vi "Client_Create.vi"(5 "Engine Factory":refnum<class "EngineFactory.lvclass">, 11 "Error In":errorcluster) -> (4 "reference out":refnum<class "Client.lvclass">, 15 "Error Out":errorcluster)   [LabVIEW 2024, in "Client.lvclass"]
uses:
  Client.lvclass/Client.ctl
  Client.lvclass
  Factory Folder/EngineFactory/EngineFactory.lvclass
panel:
  # "Connector Pane"
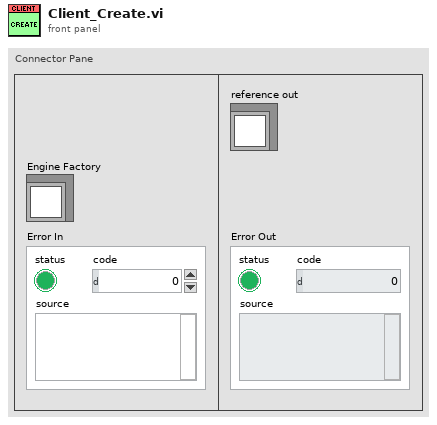
[diagram p1: front panel]
types:
  T1 = typedef "Client.lvclass/ObjectAttributes.ctl" = cluster{"Engine Factory":refnum<class "EngineFactory.lvclass">}
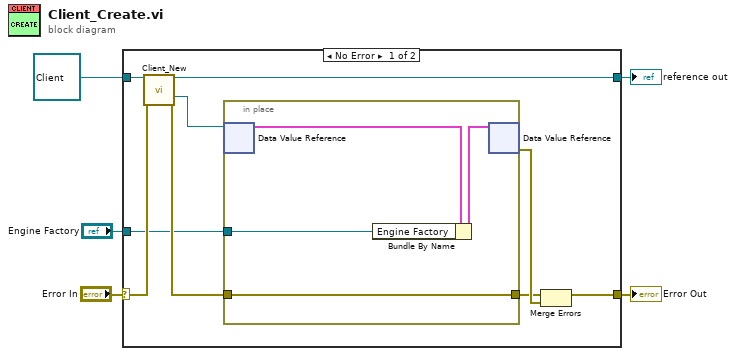
[diagram p0: block diagram]
diagram:
  n1 = case shown="No Error" "Error In" {
    selector: "Error In" -> [w13 w20]
    tunnel: [w7 w20] -> w4
    tunnel: refnum<class "Client.lvclass"> refnum ("reference in") -> [w14 w19]
    tunnel: [w12 w19] -> w2
    tunnel: "Engine Factory" -> [w6 _]
    frame No Error {
      n2 = call "Client_New.vi"("reference in"=w14, "Error In"=w13) -> ("reference out"=w12:refnum<class "Client.lvclass">, "DVRRefOut"=w10:refnum<data-value>, "Error Out"=w9:errorcluster)  [unwired: 10 in, 1 out]
      n3 = in-place {
        in-place-border: w9 -> [w16]
        in-place-border: [w16] -> w8
        in-place-border: w6 -> [w15]
        n4 = in-place-dvr #1(w10) -> (w17:T1)  [unwired: 1 out]
        n5 = Bundle By Name(cluster=w17, "Engine Factory"=w15) -> (w18:T1)
        n6 = in-place-dvr #1(w18) -> (w11:errorcluster)  [unwired: 1 out]
      }
      n7 = Merge Errors(w8, w11) -> (w7:errorcluster)
    }
    frame Error {
      # "VI-TechBaseTemplate_Simple_4x4x4"
    }
  }
  "Error Out" <- w4
  "reference out" <- w2
